vi "systeme de stockage et assemblage des pieces.vi"() -> ()   [LabVIEW 2018]
uses:
  <vilib>/NI/Modbus Library/API/Wrapper/Create TCP Master.vi
  <vilib>/NI/Modbus Library/API/Master/Modbus Master.lvclass
  <vilib>/NI/Modbus Library/API/Wrapper/API Main.lvlib
panel:
  in  "blue lid":bool
  in  "Metal lid":bool
  in  "Start":bool
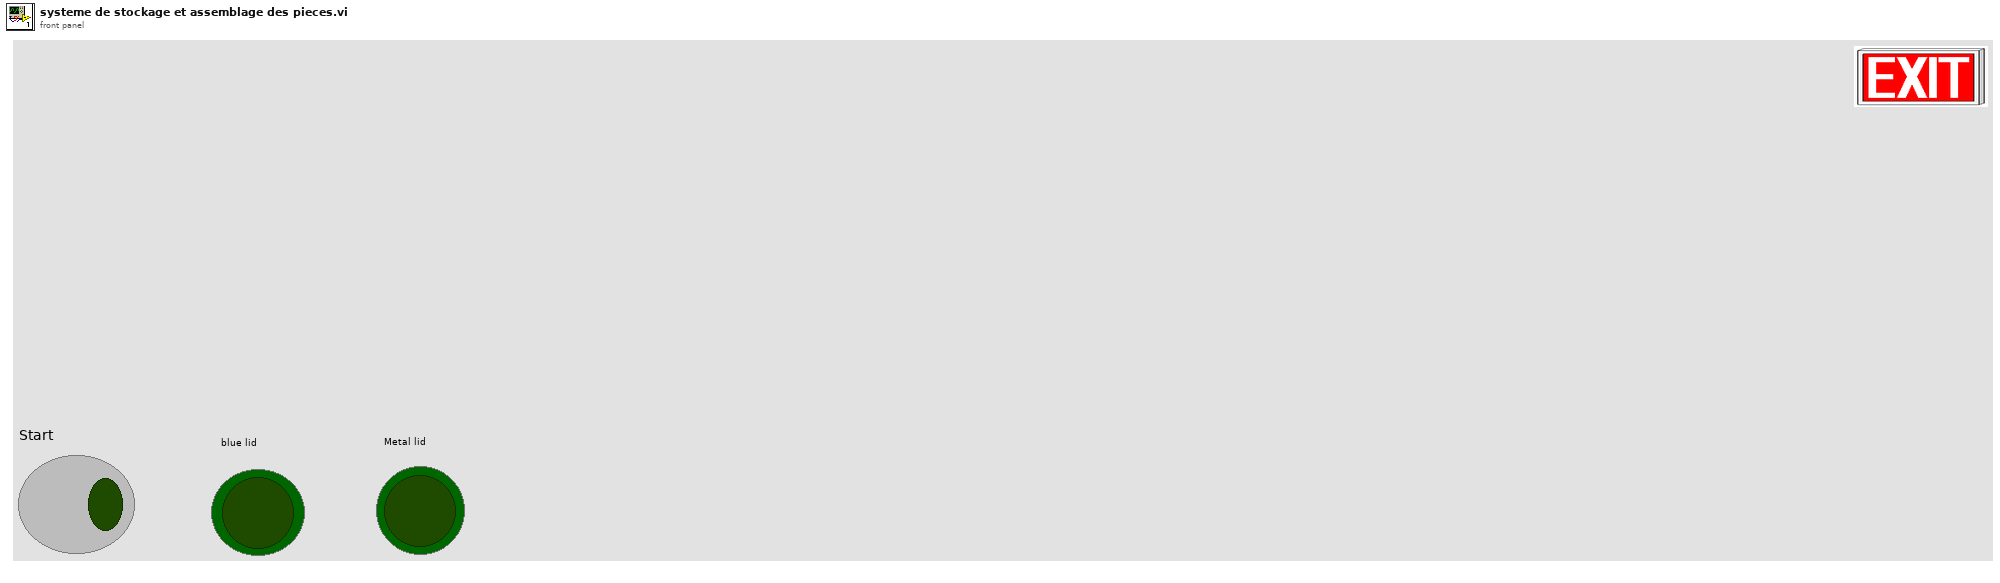
[diagram p1: front panel]
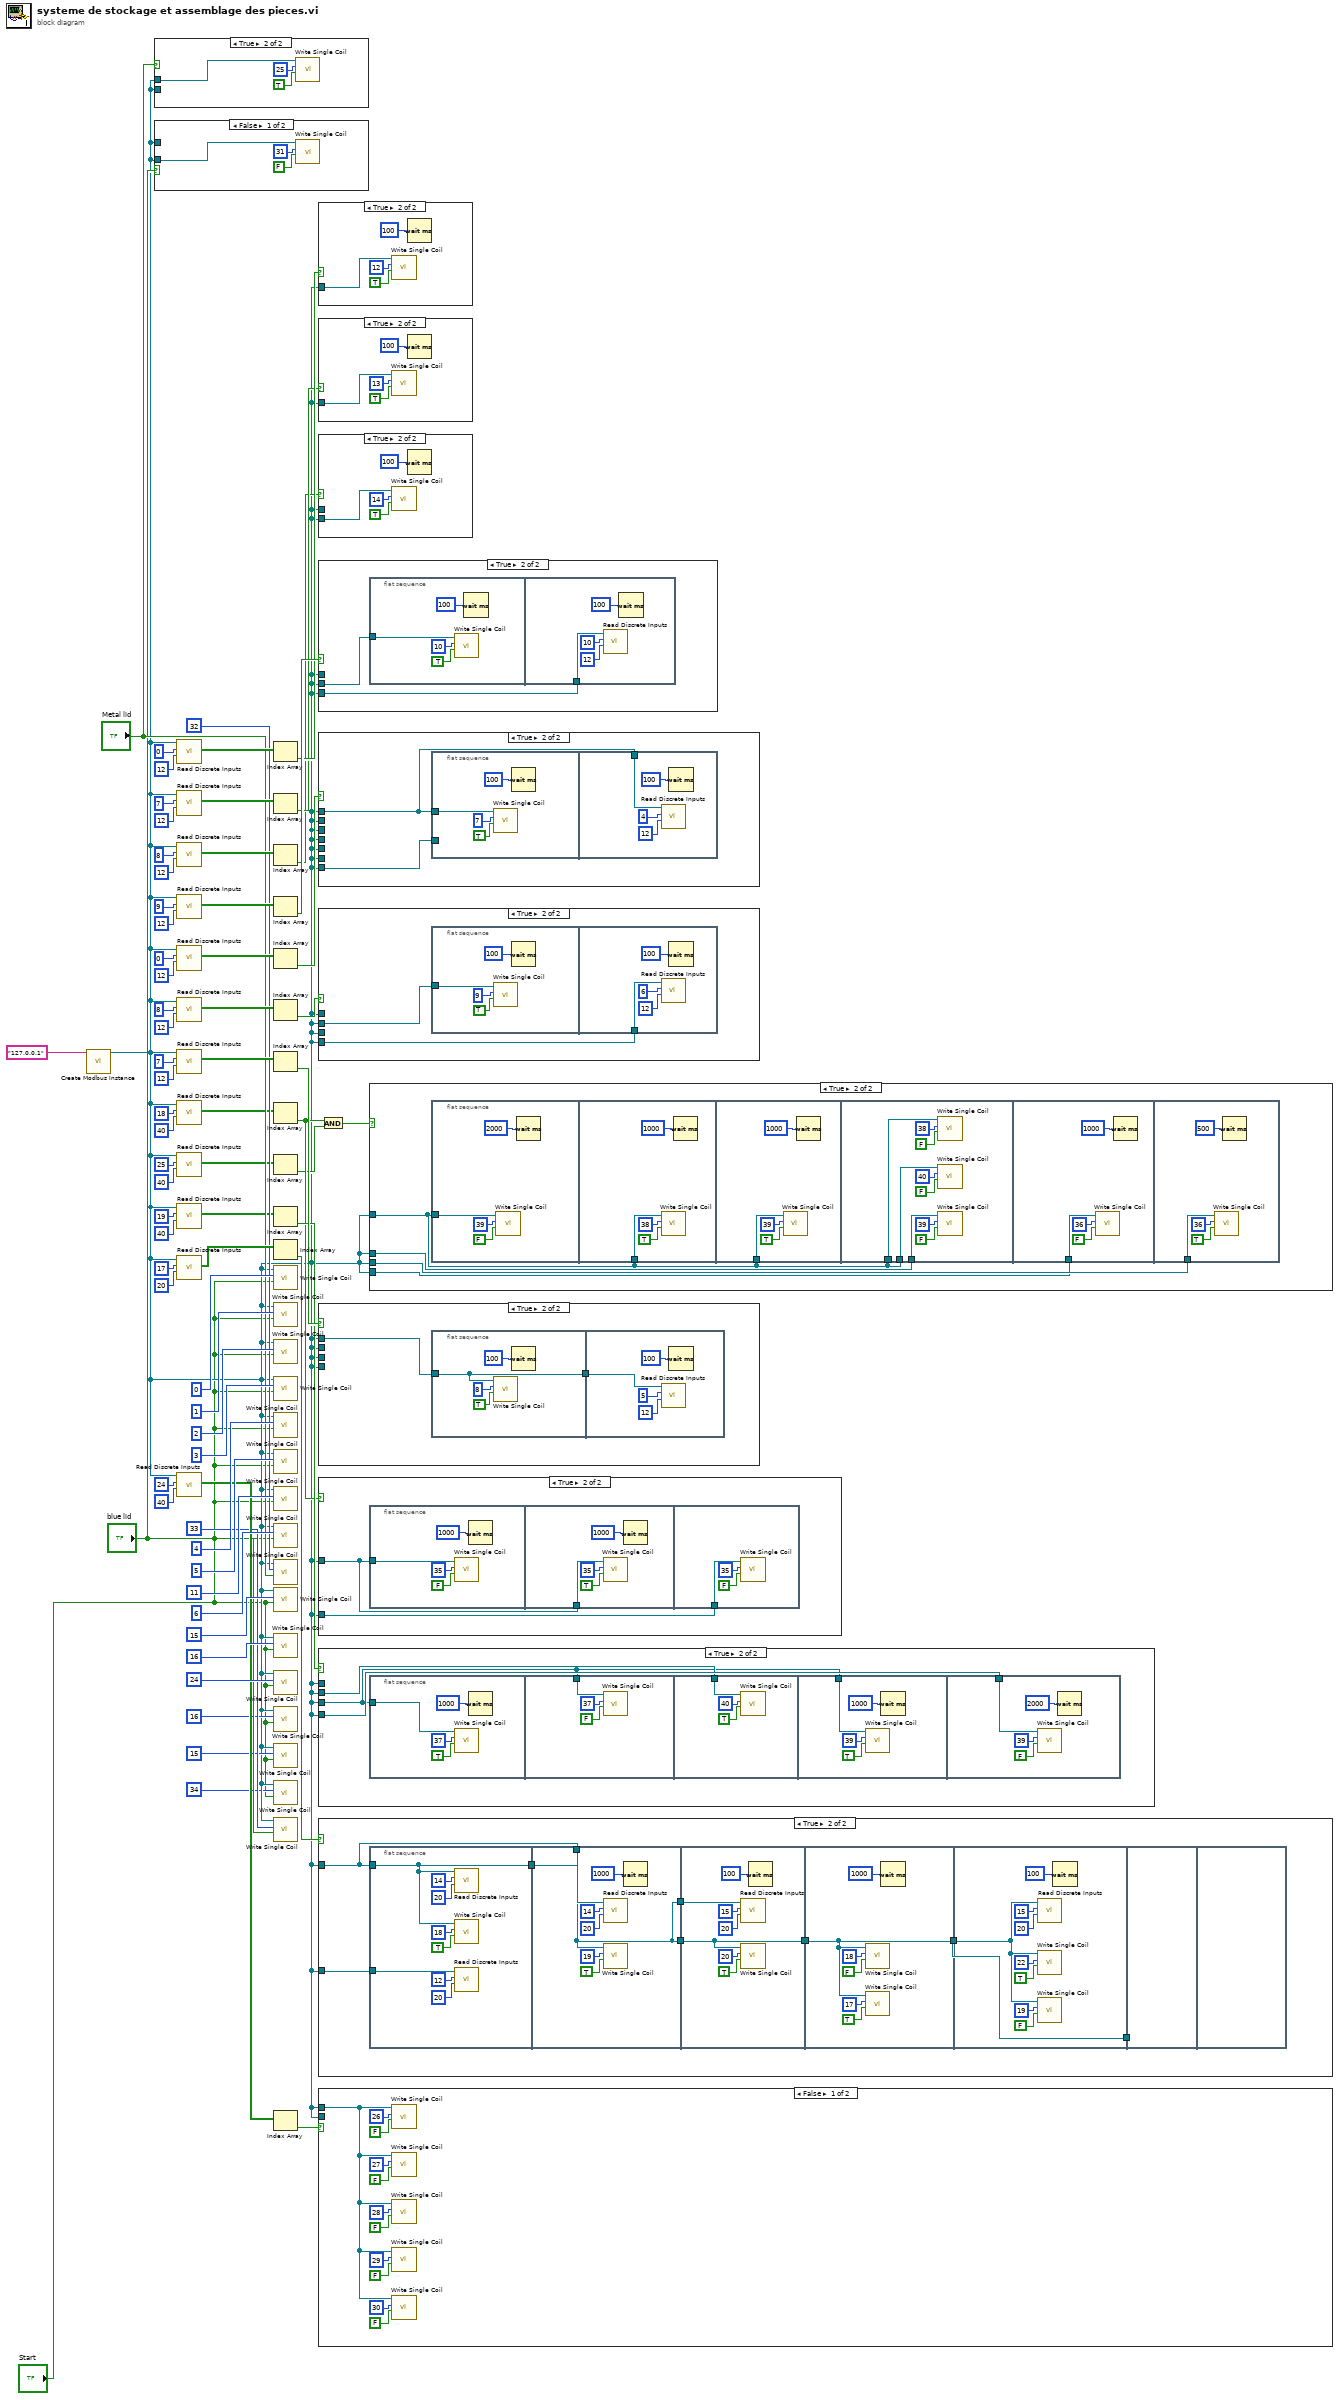
[diagram p0: block diagram]
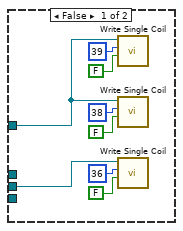
[diagram p2: hidden frame]
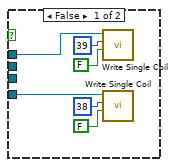
[diagram p3: hidden frame]
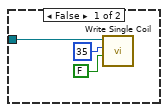
[diagram p4: hidden frame]
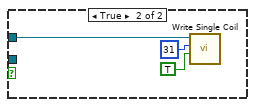
[diagram p5: hidden frame]
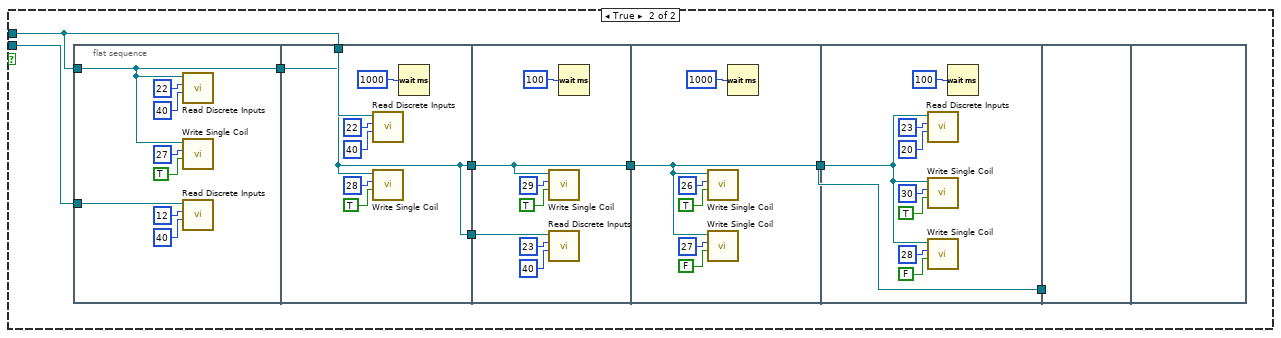
[diagram p6: hidden frame]
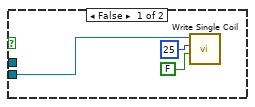
[diagram p7: hidden frame]
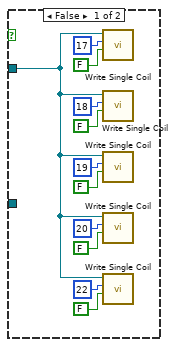
[diagram p8: hidden frame]
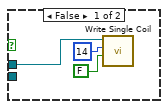
[diagram p9: hidden frame]
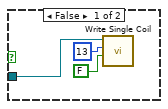
[diagram p10: hidden frame]
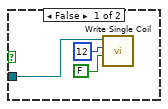
[diagram p11: hidden frame]
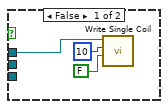
[diagram p12: hidden frame]
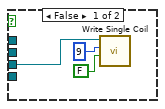
[diagram p13: hidden frame]
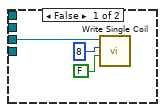
[diagram p14: hidden frame]
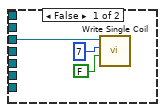
[diagram p15: hidden frame]
diagram:
  n1 = call-poly <vilib>:"Create Modbus Instance.vi"("address"="127.0.0.1") -> ("TCP master instance"=w3:refnum<class "Modbus Master.lvclass">)  [unwired: 9 in, 1 out]
  n2 = case shown="True" "Metal lid" {
    tunnel: w3 -> [_ w74]
    tunnel: w3 -> [w72 _]
    frame False {
      n3 = call-dynamic "Write Single Coil.vi"("coil to write"=FALSE, "address"=u16 25, "Modbus master in"=w72) -> ()  [unwired: 7 in, 2 out]
    }
    frame True {
      n4 = call-dynamic "Write Single Coil.vi"("coil to write"=TRUE, "address"=u16 25, "Modbus master in"=w74) -> ()  [unwired: 7 in, 2 out]
    }
  }
  n5 = case shown="False" "blue lid" {
    tunnel: w3 -> [_ w80]
    tunnel: w3 -> [w78 _]
    frame False {
      n6 = call-dynamic "Write Single Coil.vi"("coil to write"=FALSE, "address"=u16 31, "Modbus master in"=w78) -> ()  [unwired: 7 in, 2 out]
    }
    frame True {
      n7 = call-dynamic "Write Single Coil.vi"("coil to write"=TRUE, "address"=u16 31, "Modbus master in"=w80) -> ()  [unwired: 7 in, 2 out]
    }
  }
  n8 = call-dynamic "Read Discrete Inputs.vi"("number of inputs"=u16 12, "starting address"=u16 0, "Modbus master in"=w3) -> ("discrete inputs"=w43:bool[])  [unwired: 6 in, 2 out]
  n9 = call-dynamic "Read Discrete Inputs.vi"("number of inputs"=u16 12, "starting address"=u16 7, "Modbus master in"=w3) -> ("discrete inputs"=w39:bool[])  [unwired: 6 in, 2 out]
  n10 = call-dynamic "Read Discrete Inputs.vi"("number of inputs"=u16 12, "starting address"=u16 8, "Modbus master in"=w3) -> ("discrete inputs"=w35:bool[])  [unwired: 6 in, 2 out]
  n11 = call-dynamic "Read Discrete Inputs.vi"("number of inputs"=u16 12, "starting address"=u16 9, "Modbus master in"=w3) -> ("discrete inputs"=w49:bool[])  [unwired: 6 in, 2 out]
  n12 = call-dynamic "Read Discrete Inputs.vi"("number of inputs"=u16 12, "starting address"=u16 0, "Modbus master in"=w3) -> ("discrete inputs"=w61:bool[])  [unwired: 6 in, 2 out]
  n13 = call-dynamic "Read Discrete Inputs.vi"("number of inputs"=u16 12, "starting address"=u16 8, "Modbus master in"=w3) -> ("discrete inputs"=w57:bool[])  [unwired: 6 in, 2 out]
  n14 = call-dynamic "Read Discrete Inputs.vi"("number of inputs"=u16 12, "starting address"=u16 7, "Modbus master in"=w3) -> ("discrete inputs"=w53:bool[])  [unwired: 6 in, 2 out]
  n15 = call-dynamic "Read Discrete Inputs.vi"("number of inputs"=u16 40, "starting address"=u16 18, "Modbus master in"=w3) -> ("discrete inputs"=w15:bool[])  [unwired: 6 in, 2 out]
  n16 = call-dynamic "Read Discrete Inputs.vi"("number of inputs"=u16 40, "starting address"=u16 25, "Modbus master in"=w3) -> ("discrete inputs"=w9:bool[])  [unwired: 6 in, 2 out]
  n17 = call-dynamic "Read Discrete Inputs.vi"("number of inputs"=u16 40, "starting address"=u16 19, "Modbus master in"=w3) -> ("discrete inputs"=w12:bool[])  [unwired: 6 in, 2 out]
  n18 = call-dynamic "Read Discrete Inputs.vi"("number of inputs"=u16 20, "starting address"=u16 17, "Modbus master in"=w3) -> ("discrete inputs"=w31:bool[])  [unwired: 6 in, 2 out]
  n19 = call-dynamic "Read Discrete Inputs.vi"("number of inputs"=u16 40, "starting address"=u16 24, "Modbus master in"=w3) -> ("discrete inputs"=w26:bool[])  [unwired: 6 in, 2 out]
  n20 = Index Array(array=w43) -> (element=w42:bool)  [unwired: 1 in]
  n21 = Index Array(array=w39) -> (element=w38:bool)  [unwired: 1 in]
  n22 = Index Array(array=w35) -> (element=w34:bool)  [unwired: 1 in]
  n23 = Index Array(array=w49) -> (element=w48:bool)  [unwired: 1 in]
  n24 = Index Array(array=w61) -> (element=w60:bool)  [unwired: 1 in]
  n25 = Index Array(array=w57) -> (element=w56:bool)  [unwired: 1 in]
  n26 = Index Array(array=w53) -> (element=w52:bool)  [unwired: 1 in]
  n27 = Index Array(array=w15) -> (element=w7:bool)  [unwired: 1 in]
  n28 = Index Array(array=w9) -> (element=w6:bool)  [unwired: 1 in]
  n29 = Index Array(array=w12) -> (element=w8:bool)  [unwired: 1 in]
  n30 = Index Array(array=w31) -> (element=w30:bool)  [unwired: 1 in]
  n31 = call-dynamic "Write Single Coil.vi"("coil to write"="Start", "address"=u16 0, "Modbus master in"=w3) -> ()  [unwired: 7 in, 2 out]
  n32 = call-dynamic "Write Single Coil.vi"("coil to write"="Start", "address"=u16 1, "Modbus master in"=w3) -> ()  [unwired: 7 in, 2 out]
  n33 = call-dynamic "Write Single Coil.vi"("coil to write"="Start", "address"=u16 2, "Modbus master in"=w3) -> ()  [unwired: 7 in, 2 out]
  n34 = call-dynamic "Write Single Coil.vi"("coil to write"="Start", "address"=u16 3, "Modbus master in"=w3) -> ()  [unwired: 7 in, 2 out]
  n35 = call-dynamic "Write Single Coil.vi"("coil to write"="Start", "address"=u16 4, "Modbus master in"=w3) -> ()  [unwired: 7 in, 2 out]
  n36 = call-dynamic "Write Single Coil.vi"("coil to write"="Start", "address"=u16 5, "Modbus master in"=w3) -> ()  [unwired: 7 in, 2 out]
  n37 = call-dynamic "Write Single Coil.vi"("coil to write"="Start", "address"=u16 11, "Modbus master in"=w3) -> ()  [unwired: 7 in, 2 out]
  n38 = call-dynamic "Write Single Coil.vi"("coil to write"="Start", "address"=u16 6, "Modbus master in"=w3) -> ()  [unwired: 7 in, 2 out]
  n39 = call-dynamic "Write Single Coil.vi"("coil to write"="Metal lid", "address"=u16 32, "Modbus master in"=w3) -> ()  [unwired: 7 in, 2 out]
  n40 = call-dynamic "Write Single Coil.vi"("coil to write"="Start", "address"=u16 15, "Modbus master in"=w3) -> ()  [unwired: 7 in, 2 out]
  n41 = call-dynamic "Write Single Coil.vi"("coil to write"="Start", "address"=u16 16, "Modbus master in"=w3) -> ()  [unwired: 7 in, 2 out]
  n42 = call-dynamic "Write Single Coil.vi"("coil to write"="Start", "address"=u16 24, "Modbus master in"=w3) -> ()  [unwired: 7 in, 2 out]
  n43 = call-dynamic "Write Single Coil.vi"("coil to write"="Start", "address"=u16 16, "Modbus master in"=w3) -> ()  [unwired: 7 in, 2 out]
  n44 = call-dynamic "Write Single Coil.vi"("coil to write"="Start", "address"=u16 15, "Modbus master in"=w3) -> ()  [unwired: 7 in, 2 out]
  n45 = call-dynamic "Write Single Coil.vi"("coil to write"="Start", "address"=u16 34, "Modbus master in"=w3) -> ()  [unwired: 7 in, 2 out]
  n46 = call-dynamic "Write Single Coil.vi"("coil to write"="blue lid", "address"=u16 33, "Modbus master in"=w3) -> ()  [unwired: 7 in, 2 out]
  n47 = Index Array(array=w26) -> (element=w25:bool)  [unwired: 1 in]
  n48 = case shown="True" w42 {
    tunnel: w3 -> [w84 w89]
    frame False {
      n49 = call-dynamic "Write Single Coil.vi"("coil to write"=FALSE, "address"=u16 12, "Modbus master in"=w84) -> ()  [unwired: 7 in, 2 out]
    }
    frame True {
      n50 = call-dynamic "Write Single Coil.vi"("coil to write"=TRUE, "address"=u16 12, "Modbus master in"=w89) -> ()  [unwired: 7 in, 2 out]
      n51 = Wait (ms)(milliseconds to wait=u32 100) -> ()  [unwired: 1 out]
    }
  }
  n52 = case shown="True" w38 {
    tunnel: w3 -> [w90 w93]
    frame False {
      n53 = call-dynamic "Write Single Coil.vi"("coil to write"=FALSE, "address"=u16 13, "Modbus master in"=w90) -> ()  [unwired: 7 in, 2 out]
    }
    frame True {
      n54 = call-dynamic "Write Single Coil.vi"("coil to write"=TRUE, "address"=u16 13, "Modbus master in"=w93) -> ()  [unwired: 7 in, 2 out]
      n55 = Wait (ms)(milliseconds to wait=u32 100) -> ()  [unwired: 1 out]
    }
  }
  n56 = case shown="True" w34 {
    tunnel: w3 -> [_ w100]
    tunnel: w3 -> [w97 _]
    frame False {
      n57 = call-dynamic "Write Single Coil.vi"("coil to write"=FALSE, "address"=u16 14, "Modbus master in"=w97) -> ()  [unwired: 7 in, 2 out]
    }
    frame True {
      n58 = call-dynamic "Write Single Coil.vi"("coil to write"=TRUE, "address"=u16 14, "Modbus master in"=w100) -> ()  [unwired: 7 in, 2 out]
      n59 = Wait (ms)(milliseconds to wait=u32 100) -> ()  [unwired: 1 out]
    }
  }
  n60 = case shown="True" w48 {
    tunnel: w3 -> [_ w108]
    tunnel: w3 -> [_ w107]
    tunnel: w3 -> [w106 _]
    frame False {
      n61 = call-dynamic "Write Single Coil.vi"("coil to write"=FALSE, "address"=u16 10, "Modbus master in"=w106) -> ()  [unwired: 7 in, 2 out]
    }
    frame True {
      n62 = flat-sequence {
        tunnel: w108 -> [w111]
        tunnel: w107 -> [w115]
        frame #0 {
          n63 = call-dynamic "Write Single Coil.vi"("coil to write"=TRUE, "address"=u16 10, "Modbus master in"=w111) -> ()  [unwired: 7 in, 2 out]
          n64 = Wait (ms)(milliseconds to wait=u32 100) -> ()  [unwired: 1 out]
        }
        frame #1 {
          n65 = call-dynamic "Read Discrete Inputs.vi"("number of inputs"=u16 12, "starting address"=u16 10, "Modbus master in"=w115) -> ()  [unwired: 6 in, 3 out]
          n66 = Wait (ms)(milliseconds to wait=u32 100) -> ()  [unwired: 1 out]
        }
      }
    }
  }
  n67 = case shown="True" w60 {
    tunnel: w3 -> [_ _]
    tunnel: w3 -> [_ _]
    tunnel: w3 -> [_ w121]
    tunnel: w3 -> [_ w120]
    tunnel: w3 -> [_ _]
    tunnel: w3 -> [_ _]
    tunnel: w3 -> [w119 _]
    frame False {
      n68 = call-dynamic "Write Single Coil.vi"("coil to write"=FALSE, "address"=u16 7, "Modbus master in"=w119) -> ()  [unwired: 7 in, 2 out]
    }
    frame True {
      n69 = flat-sequence {
        tunnel: w121 -> [_]
        tunnel: w120 -> [w123]
        tunnel: w120 -> [w129]
        frame #0 {
          n70 = call-dynamic "Write Single Coil.vi"("coil to write"=TRUE, "address"=u16 7, "Modbus master in"=w123) -> ()  [unwired: 7 in, 2 out]
          n71 = Wait (ms)(milliseconds to wait=u32 100) -> ()  [unwired: 1 out]
        }
        frame #1 {
          n72 = call-dynamic "Read Discrete Inputs.vi"("number of inputs"=u16 12, "starting address"=u16 4, "Modbus master in"=w129) -> ()  [unwired: 6 in, 3 out]
          n73 = Wait (ms)(milliseconds to wait=u32 100) -> ()  [unwired: 1 out]
        }
      }
    }
  }
  n74 = case shown="True" w56 {
    tunnel: w3 -> [_ w134]
    tunnel: w3 -> [_ w133]
    tunnel: w3 -> [w130 _]
    tunnel: w3 -> [_ _]
    frame False {
      n75 = call-dynamic "Write Single Coil.vi"("coil to write"=FALSE, "address"=u16 9, "Modbus master in"=w130) -> ()  [unwired: 7 in, 2 out]
    }
    frame True {
      n76 = flat-sequence {
        tunnel: w134 -> [w138]
        tunnel: w133 -> [w141]
        frame #0 {
          n77 = call-dynamic "Write Single Coil.vi"("coil to write"=TRUE, "address"=u16 9, "Modbus master in"=w138) -> ()  [unwired: 7 in, 2 out]
          n78 = Wait (ms)(milliseconds to wait=u32 100) -> ()  [unwired: 1 out]
        }
        frame #1 {
          n79 = call-dynamic "Read Discrete Inputs.vi"("number of inputs"=u16 12, "starting address"=u16 6, "Modbus master in"=w141) -> ()  [unwired: 6 in, 3 out]
          n80 = Wait (ms)(milliseconds to wait=u32 100) -> ()  [unwired: 1 out]
        }
      }
    }
  }
  n81 = case shown="True" w52 {
    tunnel: w3 -> [_ w147]
    tunnel: w3 -> [_ _]
    tunnel: w3 -> [_ _]
    tunnel: w3 -> [w145 _]
    frame False {
      n82 = call-dynamic "Write Single Coil.vi"("coil to write"=FALSE, "address"=u16 8, "Modbus master in"=w145) -> ()  [unwired: 7 in, 2 out]
    }
    frame True {
      n83 = flat-sequence {
        tunnel: w147 -> [w149]
        tunnel: [w149] -> w146
        tunnel: w146 -> [w152]
        frame #0 {
          n84 = call-dynamic "Write Single Coil.vi"("coil to write"=TRUE, "address"=u16 8, "Modbus master in"=w149) -> ()  [unwired: 7 in, 2 out]
          n85 = Wait (ms)(milliseconds to wait=u32 100) -> ()  [unwired: 1 out]
        }
        frame #1 {
          n86 = call-dynamic "Read Discrete Inputs.vi"("number of inputs"=u16 12, "starting address"=u16 5, "Modbus master in"=w152) -> ()  [unwired: 6 in, 3 out]
          n87 = Wait (ms)(milliseconds to wait=u32 100) -> ()  [unwired: 1 out]
        }
      }
    }
  }
  n88 = case shown="True" w7 {
    tunnel: w3 -> [w158 w159]
    tunnel: w3 -> [_ w160]
    frame False {
      n89 = call-dynamic "Write Single Coil.vi"("coil to write"=FALSE, "address"=u16 35, "Modbus master in"=w158) -> ()  [unwired: 7 in, 2 out]
    }
    frame True {
      n90 = flat-sequence {
        tunnel: w159 -> [w161]
        tunnel: w159 -> [w165]
        tunnel: w160 -> [w169]
        frame #0 {
          n91 = call-dynamic "Write Single Coil.vi"("coil to write"=FALSE, "address"=u16 35, "Modbus master in"=w161) -> ()  [unwired: 7 in, 2 out]
          n92 = Wait (ms)(milliseconds to wait=u32 1000) -> ()  [unwired: 1 out]
        }
        frame #1 {
          n93 = call-dynamic "Write Single Coil.vi"("coil to write"=TRUE, "address"=u16 35, "Modbus master in"=w165) -> ()  [unwired: 7 in, 2 out]
          n94 = Wait (ms)(milliseconds to wait=u32 1000) -> ()  [unwired: 1 out]
        }
        frame #2 {
          n95 = call-dynamic "Write Single Coil.vi"("coil to write"=FALSE, "address"=u16 35, "Modbus master in"=w169) -> ()  [unwired: 7 in, 2 out]
        }
      }
    }
  }
  n96 = case shown="True" w8 {
    tunnel: w3 -> [w175 _]
    tunnel: w3 -> [w172 w180]
    tunnel: w3 -> [_ w179]
    tunnel: w3 -> [_ w178]
    frame False {
      n97 = call-dynamic "Write Single Coil.vi"("coil to write"=FALSE, "address"=u16 39, "Modbus master in"=w175) -> ()  [unwired: 7 in, 2 out]
      n98 = call-dynamic "Write Single Coil.vi"("coil to write"=FALSE, "address"=u16 38, "Modbus master in"=w172) -> ()  [unwired: 7 in, 2 out]
    }
    frame True {
      n99 = flat-sequence {
        tunnel: w178 -> [w184]
        tunnel: w178 -> [w187]
        tunnel: w179 -> [w188]
        tunnel: w178 -> [w191]
        tunnel: w180 -> [w196]
        frame #0 {
          n100 = call-dynamic "Write Single Coil.vi"("coil to write"=TRUE, "address"=u16 37, "Modbus master in"=w184) -> ()  [unwired: 7 in, 2 out]
          n101 = Wait (ms)(milliseconds to wait=u32 1000) -> ()  [unwired: 1 out]
        }
        frame #1 {
          n102 = call-dynamic "Write Single Coil.vi"("coil to write"=FALSE, "address"=u16 37, "Modbus master in"=w187) -> ()  [unwired: 7 in, 2 out]
        }
        frame #2 {
          n103 = call-dynamic "Write Single Coil.vi"("coil to write"=TRUE, "address"=u16 40, "Modbus master in"=w188) -> ()  [unwired: 7 in, 2 out]
        }
        frame #3 {
          n104 = call-dynamic "Write Single Coil.vi"("coil to write"=TRUE, "address"=u16 39, "Modbus master in"=w191) -> ()  [unwired: 7 in, 2 out]
          n105 = Wait (ms)(milliseconds to wait=u32 1000) -> ()  [unwired: 1 out]
        }
        frame #4 {
          n106 = call-dynamic "Write Single Coil.vi"("coil to write"=FALSE, "address"=u16 39, "Modbus master in"=w196) -> ()  [unwired: 7 in, 2 out]
          n107 = Wait (ms)(milliseconds to wait=u32 2000) -> ()  [unwired: 1 out]
        }
      }
    }
  }
  n108 = case shown="True" w30 {
    tunnel: w3 -> [w199 w216]
    tunnel: w3 -> [_ w215]
    frame False {
      n109 = call-dynamic "Write Single Coil.vi"("coil to write"=FALSE, "address"=u16 17, "Modbus master in"=w199) -> ()  [unwired: 7 in, 2 out]
      n110 = call-dynamic "Write Single Coil.vi"("coil to write"=FALSE, "address"=u16 18, "Modbus master in"=w199) -> ()  [unwired: 7 in, 2 out]
      n111 = call-dynamic "Write Single Coil.vi"("coil to write"=FALSE, "address"=u16 19, "Modbus master in"=w199) -> ()  [unwired: 7 in, 2 out]
      n112 = call-dynamic "Write Single Coil.vi"("coil to write"=FALSE, "address"=u16 20, "Modbus master in"=w199) -> ()  [unwired: 7 in, 2 out]
      n113 = call-dynamic "Write Single Coil.vi"("coil to write"=FALSE, "address"=u16 22, "Modbus master in"=w199) -> ()  [unwired: 7 in, 2 out]
    }
    frame True {
      n114 = flat-sequence {
        tunnel: w216 -> [w223]
        tunnel: [w223] -> w217
        tunnel: w215 -> [w220]
        tunnel: w217 -> [w226]
        tunnel: w216 -> [w230]
        tunnel: [w226] -> w214
        tunnel: [w226] -> w213
        tunnel: w214 -> [w233]
        tunnel: w213 -> [w234]
        tunnel: [w233] -> w212
        tunnel: w212 -> [w240]
        tunnel: [w240] -> w211
        tunnel: w211 -> [w248]
        tunnel: [w248] -> w210
        tunnel: w210 -> [_]
        frame #0 {
          n115 = call-dynamic "Read Discrete Inputs.vi"("number of inputs"=u16 20, "starting address"=u16 14, "Modbus master in"=w223) -> ()  [unwired: 6 in, 3 out]
          n116 = call-dynamic "Write Single Coil.vi"("coil to write"=TRUE, "address"=u16 18, "Modbus master in"=w223) -> ()  [unwired: 7 in, 2 out]
          n117 = call-dynamic "Read Discrete Inputs.vi"("number of inputs"=u16 20, "starting address"=u16 12, "Modbus master in"=w220) -> ()  [unwired: 6 in, 3 out]
        }
        frame #1 {
          n118 = call-dynamic "Read Discrete Inputs.vi"("number of inputs"=u16 20, "starting address"=u16 14, "Modbus master in"=w230) -> ()  [unwired: 6 in, 3 out]
          n119 = call-dynamic "Write Single Coil.vi"("coil to write"=TRUE, "address"=u16 19, "Modbus master in"=w226) -> ()  [unwired: 7 in, 2 out]
          n120 = Wait (ms)(milliseconds to wait=u32 1000) -> ()  [unwired: 1 out]
        }
        frame #2 {
          n121 = call-dynamic "Read Discrete Inputs.vi"("number of inputs"=u16 20, "starting address"=u16 15, "Modbus master in"=w234) -> ()  [unwired: 6 in, 3 out]
          n122 = call-dynamic "Write Single Coil.vi"("coil to write"=TRUE, "address"=u16 20, "Modbus master in"=w233) -> ()  [unwired: 7 in, 2 out]
          n123 = Wait (ms)(milliseconds to wait=u32 100) -> ()  [unwired: 1 out]
        }
        frame #3 {
          n124 = call-dynamic "Write Single Coil.vi"("coil to write"=FALSE, "address"=u16 18, "Modbus master in"=w240) -> ()  [unwired: 7 in, 2 out]
          n125 = call-dynamic "Write Single Coil.vi"("coil to write"=TRUE, "address"=u16 17, "Modbus master in"=w240) -> ()  [unwired: 7 in, 2 out]
          n126 = Wait (ms)(milliseconds to wait=u32 1000) -> ()  [unwired: 1 out]
        }
        frame #4 {
          n127 = call-dynamic "Read Discrete Inputs.vi"("number of inputs"=u16 20, "starting address"=u16 15, "Modbus master in"=w248) -> ()  [unwired: 6 in, 3 out]
          n128 = call-dynamic "Write Single Coil.vi"("coil to write"=TRUE, "address"=u16 22, "Modbus master in"=w248) -> ()  [unwired: 7 in, 2 out]
          n129 = call-dynamic "Write Single Coil.vi"("coil to write"=FALSE, "address"=u16 19, "Modbus master in"=w248) -> ()  [unwired: 7 in, 2 out]
          n130 = Wait (ms)(milliseconds to wait=u32 100) -> ()  [unwired: 1 out]
        }
        frame #5 {
        }
        frame #6 {
        }
      }
    }
  }
  n131 = case shown="False" w25 {
    tunnel: w3 -> [w254 w271]
    tunnel: w3 -> [_ w270]
    frame False {
      n132 = call-dynamic "Write Single Coil.vi"("coil to write"=FALSE, "address"=u16 26, "Modbus master in"=w254) -> ()  [unwired: 7 in, 2 out]
      n133 = call-dynamic "Write Single Coil.vi"("coil to write"=FALSE, "address"=u16 27, "Modbus master in"=w254) -> ()  [unwired: 7 in, 2 out]
      n134 = call-dynamic "Write Single Coil.vi"("coil to write"=FALSE, "address"=u16 28, "Modbus master in"=w254) -> ()  [unwired: 7 in, 2 out]
      n135 = call-dynamic "Write Single Coil.vi"("coil to write"=FALSE, "address"=u16 29, "Modbus master in"=w254) -> ()  [unwired: 7 in, 2 out]
      n136 = call-dynamic "Write Single Coil.vi"("coil to write"=FALSE, "address"=u16 30, "Modbus master in"=w254) -> ()  [unwired: 7 in, 2 out]
    }
    frame True {
      n137 = flat-sequence {
        tunnel: w271 -> [w278]
        tunnel: [w278] -> w272
        tunnel: w270 -> [w275]
        tunnel: w272 -> [w281]
        tunnel: w271 -> [w285]
        tunnel: [w281] -> w269
        tunnel: [w281] -> w268
        tunnel: w269 -> [w288]
        tunnel: w268 -> [w289]
        tunnel: [w288] -> w267
        tunnel: w267 -> [w295]
        tunnel: [w295] -> w266
        tunnel: w266 -> [w303]
        tunnel: [w303] -> w265
        tunnel: w265 -> [_]
        frame #0 {
          n138 = call-dynamic "Read Discrete Inputs.vi"("number of inputs"=u16 40, "starting address"=u16 22, "Modbus master in"=w278) -> ()  [unwired: 6 in, 3 out]
          n139 = call-dynamic "Write Single Coil.vi"("coil to write"=TRUE, "address"=u16 27, "Modbus master in"=w278) -> ()  [unwired: 7 in, 2 out]
          n140 = call-dynamic "Read Discrete Inputs.vi"("number of inputs"=u16 40, "starting address"=u16 12, "Modbus master in"=w275) -> ()  [unwired: 6 in, 3 out]
        }
        frame #1 {
          n141 = call-dynamic "Read Discrete Inputs.vi"("number of inputs"=u16 40, "starting address"=u16 22, "Modbus master in"=w285) -> ()  [unwired: 6 in, 3 out]
          n142 = call-dynamic "Write Single Coil.vi"("coil to write"=TRUE, "address"=u16 28, "Modbus master in"=w281) -> ()  [unwired: 7 in, 2 out]
          n143 = Wait (ms)(milliseconds to wait=u32 1000) -> ()  [unwired: 1 out]
        }
        frame #2 {
          n144 = call-dynamic "Write Single Coil.vi"("coil to write"=TRUE, "address"=u16 29, "Modbus master in"=w288) -> ()  [unwired: 7 in, 2 out]
          n145 = call-dynamic "Read Discrete Inputs.vi"("number of inputs"=u16 40, "starting address"=u16 23, "Modbus master in"=w289) -> ()  [unwired: 6 in, 3 out]
          n146 = Wait (ms)(milliseconds to wait=u32 100) -> ()  [unwired: 1 out]
        }
        frame #3 {
          n147 = call-dynamic "Write Single Coil.vi"("coil to write"=TRUE, "address"=u16 26, "Modbus master in"=w295) -> ()  [unwired: 7 in, 2 out]
          n148 = call-dynamic "Write Single Coil.vi"("coil to write"=FALSE, "address"=u16 27, "Modbus master in"=w295) -> ()  [unwired: 7 in, 2 out]
          n149 = Wait (ms)(milliseconds to wait=u32 1000) -> ()  [unwired: 1 out]
        }
        frame #4 {
          n150 = call-dynamic "Read Discrete Inputs.vi"("number of inputs"=u16 20, "starting address"=u16 23, "Modbus master in"=w303) -> ()  [unwired: 6 in, 3 out]
          n151 = call-dynamic "Write Single Coil.vi"("coil to write"=TRUE, "address"=u16 30, "Modbus master in"=w303) -> ()  [unwired: 7 in, 2 out]
          n152 = call-dynamic "Write Single Coil.vi"("coil to write"=FALSE, "address"=u16 28, "Modbus master in"=w303) -> ()  [unwired: 7 in, 2 out]
          n153 = Wait (ms)(milliseconds to wait=u32 100) -> ()  [unwired: 1 out]
        }
        frame #5 {
        }
        frame #6 {
        }
      }
    }
  }
  n154 = And(x=w7, y=w6) -> (x .and. y?=w18:bool)
  n155 = case shown="True" w18 {
    tunnel: w3 -> [w312 w320]
    tunnel: w3 -> [w309 w319]
    tunnel: w3 -> [_ w318]
    tunnel: w3 -> [_ w317]
    frame False {
      n156 = call-dynamic "Write Single Coil.vi"("coil to write"=FALSE, "address"=u16 39, "Modbus master in"=w312) -> ()  [unwired: 7 in, 2 out]
      n157 = call-dynamic "Write Single Coil.vi"("coil to write"=FALSE, "address"=u16 38, "Modbus master in"=w312) -> ()  [unwired: 7 in, 2 out]
      n158 = call-dynamic "Write Single Coil.vi"("coil to write"=FALSE, "address"=u16 36, "Modbus master in"=w309) -> ()  [unwired: 7 in, 2 out]
    }
    frame True {
      n159 = flat-sequence {
        tunnel: w320 -> [w322]
        tunnel: w320 -> [w326]
        tunnel: w320 -> [w330]
        tunnel: w320 -> [w339]
        tunnel: w320 -> [w336]
        tunnel: w317 -> [w333]
        tunnel: w318 -> [w343]
        tunnel: w319 -> [w347]
        frame #0 {
          n160 = call-dynamic "Write Single Coil.vi"("coil to write"=FALSE, "address"=u16 39, "Modbus master in"=w322) -> ()  [unwired: 7 in, 2 out]
          n161 = Wait (ms)(milliseconds to wait=u32 2000) -> ()  [unwired: 1 out]
        }
        frame #1 {
          n162 = call-dynamic "Write Single Coil.vi"("coil to write"=TRUE, "address"=u16 38, "Modbus master in"=w326) -> ()  [unwired: 7 in, 2 out]
          n163 = Wait (ms)(milliseconds to wait=u32 1000) -> ()  [unwired: 1 out]
        }
        frame #2 {
          n164 = call-dynamic "Write Single Coil.vi"("coil to write"=TRUE, "address"=u16 39, "Modbus master in"=w330) -> ()  [unwired: 7 in, 2 out]
          n165 = Wait (ms)(milliseconds to wait=u32 1000) -> ()  [unwired: 1 out]
        }
        frame #3 {
          n166 = call-dynamic "Write Single Coil.vi"("coil to write"=FALSE, "address"=u16 38, "Modbus master in"=w336) -> ()  [unwired: 7 in, 2 out]
          n167 = call-dynamic "Write Single Coil.vi"("coil to write"=FALSE, "address"=u16 40, "Modbus master in"=w339) -> ()  [unwired: 7 in, 2 out]
          n168 = call-dynamic "Write Single Coil.vi"("coil to write"=FALSE, "address"=u16 39, "Modbus master in"=w333) -> ()  [unwired: 7 in, 2 out]
        }
        frame #4 {
          n169 = call-dynamic "Write Single Coil.vi"("coil to write"=FALSE, "address"=u16 36, "Modbus master in"=w343) -> ()  [unwired: 7 in, 2 out]
          n170 = Wait (ms)(milliseconds to wait=u32 1000) -> ()  [unwired: 1 out]
        }
        frame #5 {
          n171 = call-dynamic "Write Single Coil.vi"("coil to write"=TRUE, "address"=u16 36, "Modbus master in"=w347) -> ()  [unwired: 7 in, 2 out]
          n172 = Wait (ms)(milliseconds to wait=u32 500) -> ()  [unwired: 1 out]
        }
      }
    }
  }
